vi "Execution_SignalProcessStarted.vi"(8 "error in":errorcluster, 10 "This VI":refnum<vi>, 11 "EVE reference in":refnum<data-value>) -> (0 "error out":errorcluster)   [LabVIEW 2013, in "Process.lvclass"]
uses:
  Process.lvclass
  001 - MAIN/Class/EVE/EVE.lvclass
  001 - MAIN/Class/Messages/ProcessStartedMessage/ProcessStartedMessage.lvclass
  <vilib>/event_ctls.llb/usereventprio.ctl
  030 - EVENTS/03 - ToMessageHandlerProcess/enumMessageCriticity.ctl
  001 - MAIN/Class/Messages/ProcessStartedMessage/ProcessStartState.ctl
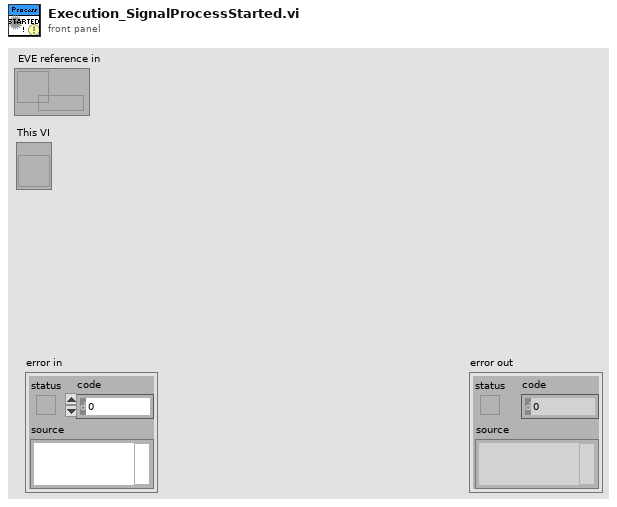
[diagram p1: front panel]
types:
  T1 = typedef "ProcessStartedMessage.lvclass/ProcessStartState.ctl" = enum16{"Started", "Started with error"}
  T2 = typedef "enumMessageCriticity.ctl" = enum16{"No error", "Info", "Warning", "Error", "Fatal error"}
  T3 = typedef "usereventprio.ctl" = enum32{"high priority", "normal priority"}
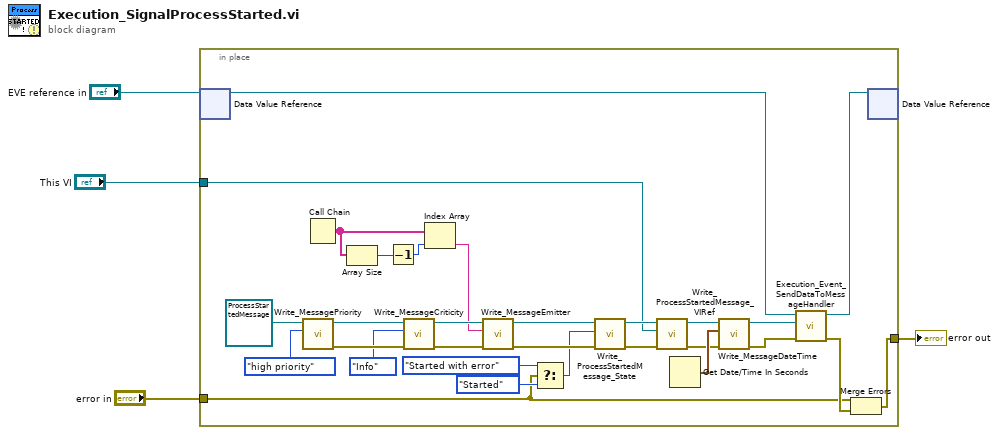
[diagram p0: block diagram]
diagram:
  n1 = in-place {
    in-place-border: "error in" -> [w6]
    in-place-border: [w5] -> w3
    in-place-border: "This VI" -> [w9]
    n2 = in-place-dvr #1("EVE reference in") -> (w33:refnum<class "EVE.lvclass">)  [unwired: 1 out]
    n3 = call-dynamic "Write_MessagePriority.vi"("user event priority"=usereventprio."high priority", "Messages in"=refnum<class "ProcessStartedMessage.lvclass"> refnum ("ProcessStartedMessage.lvclass")) -> ("error out"=w28:errorcluster, "Messages out"=w29:refnum<class "ProcessStartedMessage.lvclass">)  [unwired: 8 in]
    n4 = Call Chain() -> (call chain=w21:string[])
    n5 = Array Size(array=w21) -> (size(s)=w20:i32)
    n6 = Decrement(x=w20) -> (x-1=w19:i32)
    n7 = call-dynamic "Write_MessageCriticity.vi"("error in (no error)"=w28, "Criticity"=enumMessageCriticity."Info", "Messages in"=w29) -> ("error out"=w22:errorcluster, "Messages out"=w23:refnum<class "ProcessStartedMessage.lvclass">)  [unwired: 7 in]
    n8 = Index Array(array=w21, index=w19) -> (element=w18:string)
    n9 = call-dynamic "Write_MessageEmitter.vi"("error in (no error)"=w22, "Emitter"=w18, "Messages in"=w23) -> ("error out"=w13:errorcluster, "Messages out"=w15:refnum<class "ProcessStartedMessage.lvclass">)  [unwired: 7 in]
    n10 = Select(t=ProcessStartState."Started with error" ("State"), s=w6, f=ProcessStartState."Started") -> (s? t:f=w8:T1)
    n11 = call-dynamic "Write_ProcessStartedMessage_State.vi"("error in (no error)"=w13, "State"=w8, "ProcessStartedMessage in"=w15) -> ("error out"=w16:errorcluster, "ProcessStartedMessage out"=w17:refnum<class "ProcessStartedMessage.lvclass">)  [unwired: 7 in]
    n12 = call-dynamic "Write_ProcessStartedMessage_VIRef.vi"("error in (no error)"=w16, "VI Refnum"=w9, "ProcessStartedMessage in"=w17) -> ("error out"=w12:errorcluster, "ProcessStartedMessage out"=w14:refnum<class "ProcessStartedMessage.lvclass">)  [unwired: 7 in]
    n13 = Get Date/Time In Seconds() -> (seconds since 1Jan1904=w24:timestamp)
    n14 = call-dynamic "Write_MessageDateTime.vi"("error in (no error)"=w12, "date / time"=w24, "Messages in"=w14) -> ("error out"=w25:errorcluster, "Messages out"=w26:refnum<class "ProcessStartedMessage.lvclass">)  [unwired: 7 in]
    n15 = call-dynamic "Execution_Event_SendDataToMessageHandler.vi"("error in (no error)"=w25, "Message"=w26, "EVE in"=w33) -> ("error out"=w7:errorcluster, "EVE out"=w32:refnum<class "EVE.lvclass">)  [unwired: 7 in]
    n16 = Merge Errors(w6, w7) -> (w5:errorcluster)
    n17 = in-place-dvr #1(w32) -> ()  [unwired: 2 out]
  }
  "error out" <- w3
